vi "CH_LM App FGV DevicesInUse.vi"(0 "Device Array":T1[](array[typedef]), 1 "set? (F)":bool) -> (2 "Device Array":T1[](array[typedef]))   [LabVIEW 2012, in "CH_LM App.lvlib"]
doc: "This FGV stores the LabMax meters in use."
uses:
  CH_LM App.lvlib
  CH_LM App Meter.ctl
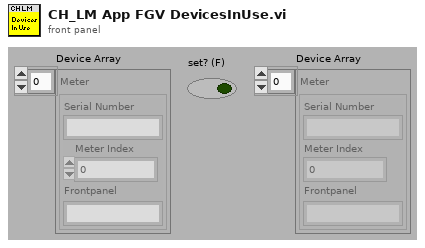
[diagram p1: front panel]
types:
  T1 = typedef "CH_LM App.lvlib/CH_LM App Meter.ctl" = cluster{"Serial Number":string, "Meter Index":i32, "Frontpanel":string}
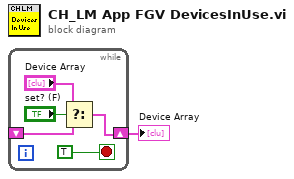
[diagram p0: block diagram]
diagram:
  n1 = while {
    shift-right: [w3] -> w1
    shift-left: _ -> [w2]
    stop <- TRUE stop-if-true
    n2 = Select(t="Device Array", s="set? (F)", f=w2) -> (s? t:f=w3:T1[])
  }
  "Device Array" <- w1
